vi "try repair.vi"(8 "error in":errorcluster, 11 "configuration in":refnum<class "NISE_CEF_serializable configuration.lvclass">) -> (0 "error out":errorcluster, 1 "change occurred":bool, 2 "repair report":string, 3 "configuration out":refnum<class "NISE_CEF_serializable configuration.lvclass">)   [LabVIEW 2013, in "NISE_CEF_serializable configuration.lvclass"]
uses:
  NISE_CEF_serializable configuration.lvclass
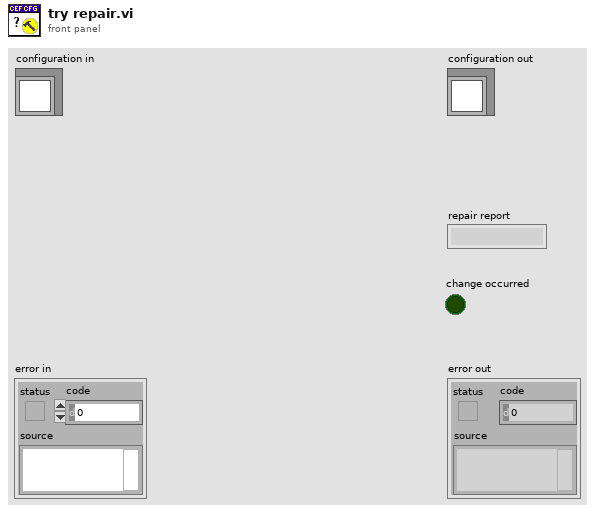
[diagram p1: front panel]
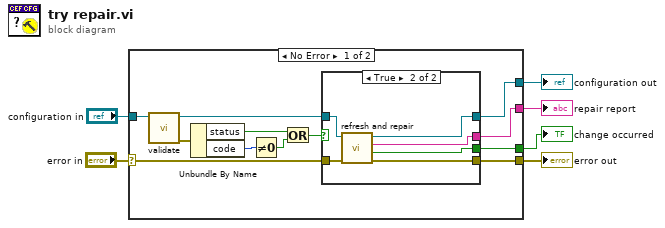
[diagram p0: block diagram]
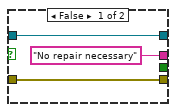
[diagram p2: hidden frame]
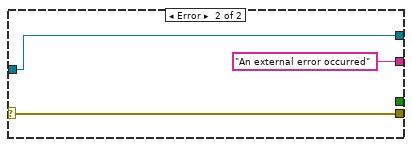
[diagram p3: hidden frame]
diagram:
  n1 = case shown="No Error" "error in" {
    selector: "error in" -> [w9 w30]
    tunnel: [w8 w30] -> w5
    tunnel: [w11 w29] -> w3
    tunnel: "configuration in" -> [w18 w29]
    tunnel: [w10 "An external error occurred"] -> w2
    tunnel: [w7 _] -> w1
    frame No Error {
      n2 = call-dynamic "validate.vi"("configuration in"=w18) -> ("error out"=w17:errorcluster, "configuration out"=w12:refnum<class "NISE_CEF_serializable configuration.lvclass">)  [unwired: 9 in]
      n3 = Unbundle By Name(w17) -> ("status"=w14:bool, "code"=w16:i32)
      n4 = Not Equal To 0?(x=w16) -> (x != 0?=w15:bool)
      n5 = Or(x=w14, y=w15) -> (x .or. y?=w13:bool)
      n6 = case shown="True" w13 {
        tunnel: w12 -> [w21 w27]
        tunnel: [w21 w23] -> w11
        tunnel: ["No repair necessary" w24] -> w10
        tunnel: w9 -> [w19 w26]
        tunnel: [w19 w25] -> w8
        tunnel: [_ w22] -> w7
        frame False {
        }
        frame True {
          n7 = call-dynamic "refresh and repair.vi"("error in"=w26, "configuration in"=w27) -> ("error out"=w25:errorcluster, "data changed?"=w22:bool, "repair report"=w24:string, "configuration out"=w23:refnum<class "NISE_CEF_serializable configuration.lvclass">)  [unwired: 6 in]
        }
      }
    }
    frame Error {
    }
  }
  "error out" <- w5
  "configuration out" <- w3
  "repair report" <- w2
  "change occurred" <- w1
